vi "3D Viewer - Test.vi"() -> ()   [LabVIEW 2017]
panel:
  in  "Angle Z":sgl
  in  "Angle Y":sgl
  in  "Angle X":sgl
  in  "stop":bool
  out "3D Picture":refnum<vi>(3d-picture)
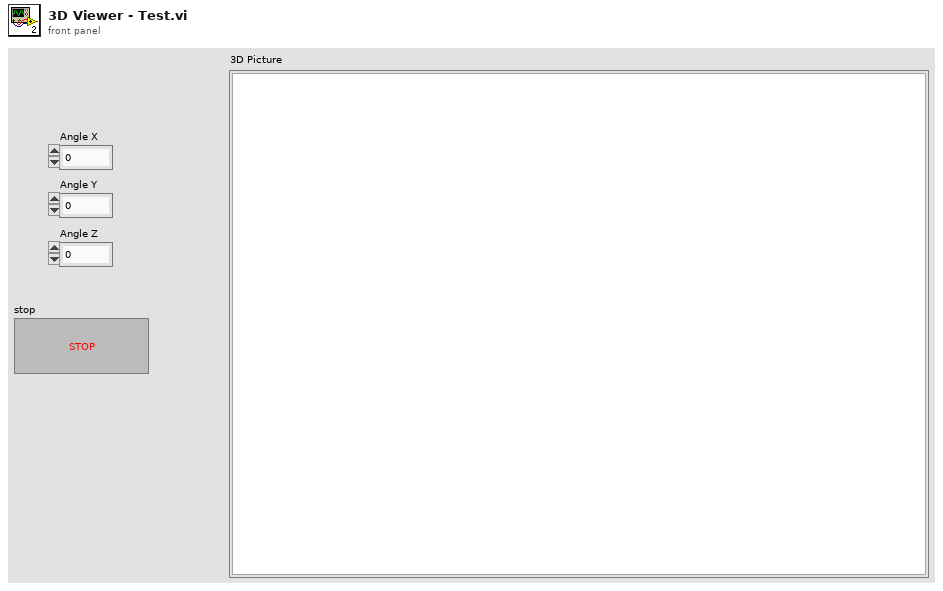
[diagram p1: front panel]
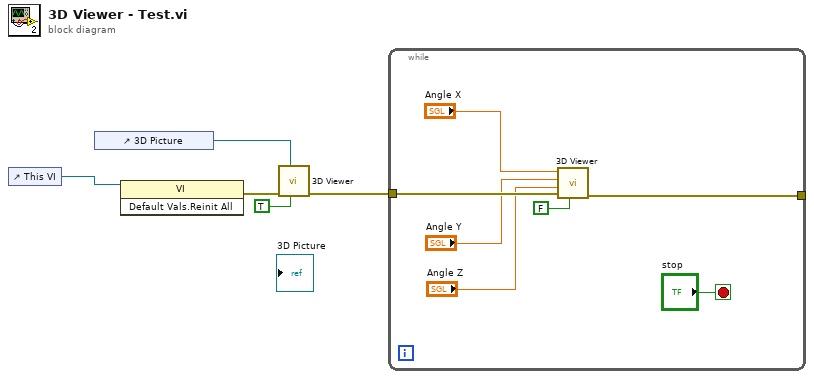
[diagram p0: block diagram]
diagram:
  n1 = control-ref of="This VI"() -> (w2:refnum<vi>)
  n2 = control-ref of="3D Picture"() -> (w5:refnum<vi>)
  n3 = invoke class="VI" method="Default Vals.Reinit All"(reference=w2) -> (error out=w3:errorcluster)  [unwired: 2 in, 2 out]
  n4 = call "3D Viewer.vi"("Initialize ?"=TRUE, "3D View Image"=w5, "error in (no error)"=w3) -> ("error out"=w1:errorcluster)  [unwired: 7 in, 1 out]
  n5 = while {
    tunnel: w1 -> [w12]
    tunnel: [w10] -> _
    stop <- "stop" stop-if-true
    n6 = call "3D Viewer.vi"("Initialize ?"=FALSE, "error in (no error)"=w12, "Angle Z"="Angle Z", "Angle Y"="Angle Y", "Angle X"="Angle X") -> ("error out"=w10:errorcluster)  [unwired: 5 in, 1 out]
  }
